vi "util_manual_transition.vi"(7 "references":T1, 8 "error in (no error)":errorcluster, 11 "data":variant) -> (0 "error out":errorcluster)   [LabVIEW 2015, in "lv-recipe-machine.lvlib"]
uses:
  lv-recipe-machine.lvlib
  _controls/references.ctl
  private/_controls/input.ctl
  private/_controls/input_command.ctl
  private/_controls/output.ctl
  private/_controls/data.ctl
  _controls/configuration.ctl
  private/_controls/recipe_data.ctl
  _controls/mode.ctl
  _controls/manual_state.ctl
  _controls/automatic_state.ctl
  _controls/recipe_step.ctl
  <userlib>/antonio-alexander/lv-waitgroup/public/_controls/api_waitgroup.ctl
  _controls/transition.ctl
  _controls/change.ctl
  _controls/status.ctl
  <userlib>/antonio-alexander/lv-waitgroup/lv-waitgroup.lvlib
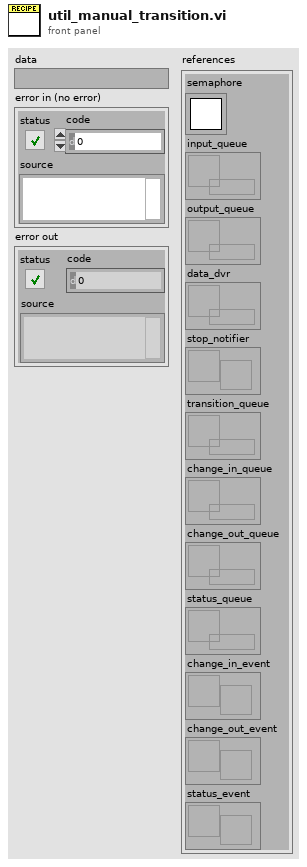
[diagram p1: front panel]
types:
  T1 = typedef "lv-recipe-machine.lvlib/references.ctl" = cluster{"semaphore":T2, "input_queue":refnum<queue>, "output_queue":refnum<queue>, "data_dvr":refnum<data-value>, "stop_notifier":refnum<notifier>, "transition_queue":refnum<queue>, "change_in_queue":refnum<queue>, "change_out_queue":refnum<queue>, "status_queue":refnum<queue>, "change_in_event":refnum<user-event>, "change_out_event":refnum<user-event>, "status_event":refnum<user-event>}
  T2 = typedef "Semaphore RefNum" = refnum<k1>
  T3 = typedef "lv-recipe-machine.lvlib/transition.ctl" = cluster{"next_step":string, "next_index":i32, "data":variant, "error":errorcluster}
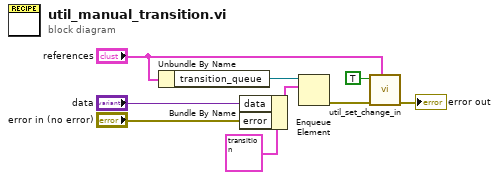
[diagram p0: block diagram]
diagram:
  n1 = Unbundle By Name("references") -> ("transition_queue"=w2:refnum<queue>)
  n2 = Bundle By Name(cluster=T3 {"next_step"="", "next_index"=0, "data"=variant, "error"={"status"=FALSE, "code"=0, "source"=""}} ("transition"), "data"="data", "error"="error in (no error)") -> (w7:T3)
  n3 = Enqueue Element(queue=w2, element=w7) -> (error out=w4:errorcluster)  [unwired: 2 in, 2 out]
  n4 = call "util_set_change_in.vi"("references"="references", "error in (no error)"=w4, "change"=TRUE) -> ("error out"=→"error out":errorcluster)  [unwired: 8 in]
